vi "parse_clz_series.vi"(11 "clz comics":T2[](array[typedef]) {"Release Date" format="%<%x>T"}) -> (3 "clz series map":map{i32, T1}(c390))   [LabVIEW 2024, in "CLZ_to_ComicVine.lvlib"]
uses:
  CLZ_to_ComicVine.lvlib
  typedefs/CLZ_comic.ctl
  typedefs/CLZ_series.ctl
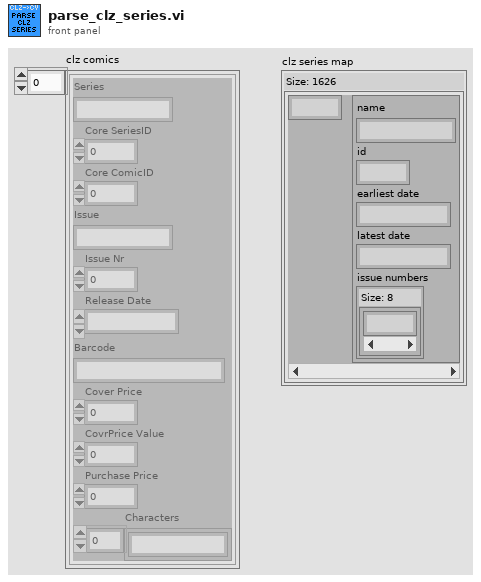
[diagram p1: front panel]
types:
  T1 = typedef "CLZ_to_ComicVine.lvlib/CLZ_series.ctl" = cluster{"name":string, "id":i32, "earliest date":timestamp, "latest date":timestamp, "issue numbers":set{i32}}
  T2 = typedef "CLZ_to_ComicVine.lvlib/CLZ_comic.ctl" = cluster{"Series":string, "Core SeriesID":i32, "Core ComicID":i32, "Issue":string, "Issue Nr":i32, "Release Date":timestamp, "Barcode":string, "Cover Price":dbl, "CovrPrice Value":dbl, "Purchase Price":dbl, "Characters":string[]}
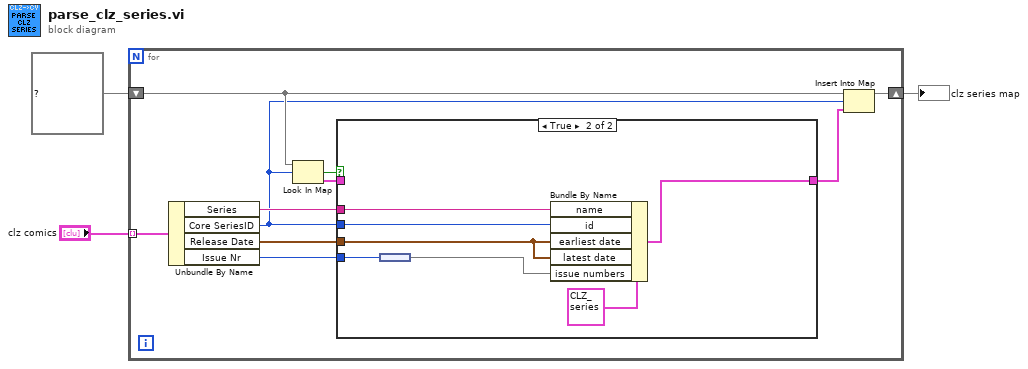
[diagram p0: block diagram]
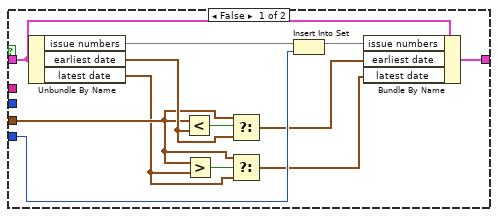
[diagram p2: hidden frame]
diagram:
  n1 = for {
    tunnel: "clz comics" -> [w13] mode=indexing
    shift-right: [w6] -> w2
    shift-left: map{i32, T1} {} ("map") -> [w9]
    n2 = Unbundle By Name(w13) -> ("Series"=w11:string, "Core SeriesID"=w8:i32, "Release Date"=w10:timestamp, "Issue Nr"=w4:i32)
    n3 = Look In Map(map=w9, key=w8) -> (key not found?=w12:bool, value=w5:T1)  [unwired: 1 in]
    n4 = case shown="True" w12 {
      tunnel: w11 -> [_ w31]
      tunnel: w8 -> [_ w30]
      tunnel: w10 -> [w17 w29]
      tunnel: [w14 w28] -> w7
      tunnel: w5 -> [w25 _]
      tunnel: w4 -> [w21 w27]
      frame False {
        n5 = Unbundle By Name(w25) -> ("issue numbers"=w24:set{i32}, "earliest date"=w20:timestamp, "latest date"=w16:timestamp)
        n6 = Less?(x=w17, y=w20) -> (x < y?=w22:bool)
        n7 = Greater?(x=w17, y=w16) -> (0:w18:bool)
        n8 = Select(t=w17, s=w22, f=w20) -> (s? t:f=w19:timestamp)
        n9 = Select(t=w17, s=w18, f=w16) -> (s? t:f=w15:timestamp)
        n10 = Insert Into Set(10:w21, 11:w24) -> (3:w23:set{i32})  [unwired: 1 out]
        n11 = Bundle By Name(cluster=w25, "issue numbers"=w23, "earliest date"=w19, "latest date"=w15) -> (w14:T1)
      }
      frame True {
        n12 = node(w27) -> (w26:set{i32})
        n13 = Bundle By Name(cluster=T1 {"name"="", "id"=0, "earliest date"=timestamp(0 s since 1904-01-01), "latest date"=timestamp(0 s since 1904-01-01), "issue numbers"={}} ("clz series"), "name"=w31, "id"=w30, "earliest date"=w29, "latest date"=w29, "issue numbers"=w26) -> (w28:T1)
      }
    }
    n14 = Insert Into Map(map in=w9, key=w8, value=w7) -> (map out=w6:map{i32, T1})  [unwired: 2 out]
  }
  "clz series map" <- w2
